vi "AVS_Register.vi"(7 "a_hWnd":i32) -> (8 "Output Value":i32)   [LabVIEW 2009]
uses:
  avaspecx64.dll
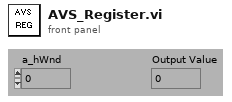
[diagram p1: front panel]
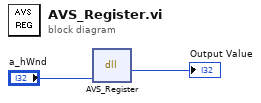
[diagram p0: block diagram]
diagram:
  n1 = dll-call lib="E:/Documents and Settings/mattc/Libraries/Avaspec_Library/trunk/demo_64bit/LabView/LabViewSingleChan/avaspecx64.dll" fn="AVS_Register"("a_hWnd"="a_hWnd") -> ("return type"=→"Output Value":i32)  [unwired: 4 in, 2 out]
